vi "Config-Chan-SMU-Sweep.vi"(0 "VISA session":refnum<visa-resource-name>, 1 "function":i32(slide) max=4 scale=0.0..4.0, 2 "I name (max 6 chars)":string, 5 "unit to configure":i32(slide) max=5 scale=0.0..5.0, 7 "series resistance *":i32(slide) max=3 scale=0.0..3.0, 9 "standby":bool, 11 "error in (no error)":errorcluster, 12 "mode":i32(slide) max=4 scale=0.0..4.0, 13 "V name (max 6 chars)":string) -> (4 "VISA resource name out":refnum<visa-resource-name>, 15 "error out":errorcluster)   [LabVIEW 2016, in "Agilent 415X Series.lvlib"]
doc: "This VI configures an SMU for SWEEP mode measurement. \n\nThis VI corresponds to the Channel Definition Page of the instrument (when Measurement Mode is SWEEP). In general, it allows every setting change that can be made via the instrument's front panel although the change may cause a setting conflict when a measurement is initialied. This VI doesnot allow (by reporting an error) setting changes that can not be made via the instrument's front panel. For example, you may not set Series Resistance for units other than SMU1, SMU2/5.\n\n** The instrument used in the development of this instrument driver does not have an Expander Unit installed. Therefore commands related to SMU5/6 have not been verified."
uses:
  Agilent 415X Series.lvlib
panel:
  # "<--->"
  # "*   The Series Resistance control is active only if UnitToConfigure is SMU1 or SMU2/SMU5 (see description)\n** This VI does NOT report all setting errors.  Error checking must be done when a measurement is initialized."
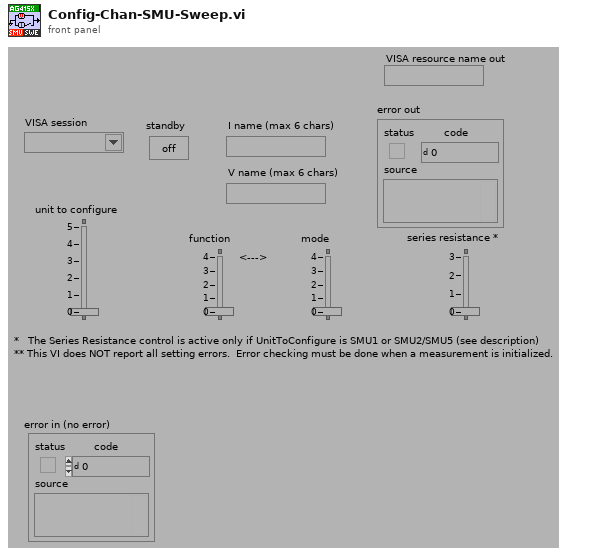
[diagram p1: front panel]
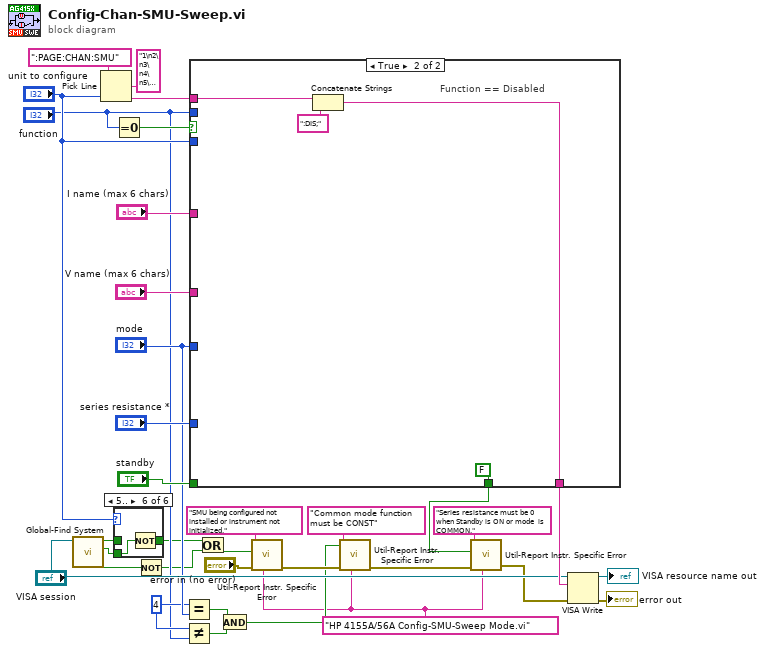
[diagram p0: block diagram]
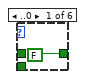
[diagram p2: hidden frame]
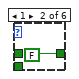
[diagram p3: hidden frame]
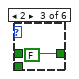
[diagram p4: hidden frame]
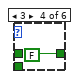
[diagram p5: hidden frame]
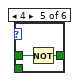
[diagram p6: hidden frame]
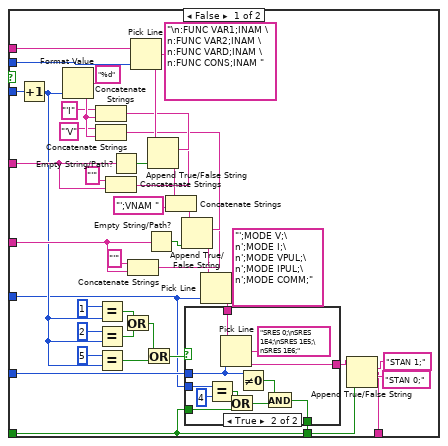
[diagram p7: hidden frame]
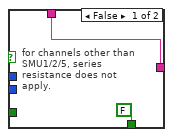
[diagram p8: hidden frame]
diagram:
  w12 = 4
  w8 = "HP 4155A/56A Config-SMU-Sweep Mode.vi"
  n1 = call "Global-Find System.vi"("VISA session"="VISA session") -> ("found"=w3:bool, "SMU6 present"=w24:bool, "SMU5 present"=w18:bool)  [unwired: 3 in, 5 out]
  n2 = Pick Line(string ("")=":PAGE:CHAN:SMU", multi-line string="1\n2\n3\n4\n5\n6", line index="unit to configure") -> (output string=w32:string)
  n3 = Equal To 0?(x="function") -> (x = 0?=w26:bool)
  n4 = case shown="5.." "unit to configure" {
    tunnel: [FALSE FALSE FALSE FALSE w40 w42] -> w4
    tunnel: w24 -> [_ _ _ _ _ w41]
    tunnel: w18 -> [_ _ _ _ w39 _]
    frame ..0 {
    }
    frame 1 {
    }
    frame 2 {
    }
    frame 3 {
    }
    frame 4 {
      n5 = Not(x=w39) -> (.not. x?=w40:bool)
    }
    frame 5.. {
      n6 = Not(x=w41) -> (.not. x?=w42:bool)
    }
  }
  n7 = Not(x=w3) -> (.not. x?=w2:bool)
  n8 = Equal?(x=w12, y="mode") -> (x = y?=w16:bool)
  n9 = Not Equal?(x=w12, y="function") -> (x != y?=w15:bool)
  n10 = case shown="True" w26 {
    tunnel: w32 -> [w83 w101]
    tunnel: "function" -> [w80 _]
    tunnel: "unit to configure" -> [w49 _]
    tunnel: "I name (max 6 chars)" -> [w74 _]
    tunnel: "V name (max 6 chars)" -> [w65 _]
    tunnel: "mode" -> [w44 _]
    tunnel: "series resistance *" -> [w58 _]
    tunnel: "standby" -> [w45 _]
    tunnel: [w46 w99] -> w28
    tunnel: [w43 FALSE] -> w6
    frame False {
      n11 = Increment(x=w49) -> (x+1=w47:i32)
      n12 = Format Value(format string="%d", value (0)=w47) -> (output string=w78:string)  [unwired: 1 in]
      n13 = Concatenate Strings("'I", w78) -> (w75:string)
      n14 = Concatenate Strings("'V", w78) -> (w68:string)
      n15 = Equal?(x=1, y=w47) -> (x = y?=w54:bool)
      n16 = Equal?(x=2, y=w47) -> (x = y?=w53:bool)
      n17 = Equal?(x=5, y=w47) -> (x = y?=w52:bool)
      n18 = Concatenate Strings("'", w74) -> (w72:string)
      n19 = Empty String/Path?(string/path=w74) -> (empty?=w81:bool)
      n20 = Or(x=w54, y=w53) -> (x .or. y?=w51:bool)
      n21 = Concatenate Strings("'", w65) -> (w64:string)
      n22 = Pick Line(string ("")=w83, multi-line string="\n:FUNC VAR1;INAM \n:FUNC VAR2;INAM \n:FUNC VARD;INAM \n:FUNC CONS;INAM ", line index=w80) -> (output string=w82:string)
      n23 = Or(x=w51, y=w52) -> (x .or. y?=w50:bool)
      n24 = Empty String/Path?(string/path=w65) -> (empty?=w67:bool)
      n25 = Append True/False String(1:w81, 2:w72, 3:w75, 4:w82) -> (0:w71:string)
      n26 = Concatenate Strings(w71, "';VNAM ") -> (w69:string)
      n27 = Append True/False String(1:w67, 2:w64, 3:w68, 4:w69) -> (0:w62:string)
      n28 = Pick Line(string ("")=w62, multi-line string="';MODE V;\n';MODE I;\n';MODE VPUL;\n';MODE IPUL;\n';MODE COMM;", line index=w44) -> (output string=w59:string)
      n29 = case shown="True" w50 {
        tunnel: w59 -> [w86 w96]
        tunnel: w58 -> [_ w89]
        tunnel: [w86 w95] -> w57
        tunnel: w45 -> [_ w92]
        tunnel: w44 -> [_ w94]
        tunnel: [FALSE w87] -> w43
        frame False {
          # "for channels other than\nSMU1/2/5, series \nresistance does not \napply."
        }
        frame True {
          n30 = Equal?(x=w94, y=4) -> (x = y?=w91:bool)
          n31 = Pick Line(string ("")=w96, multi-line string="SRES 0;\nSRES 1E4;\nSRES 1E5;\nSRES 1E6;", line index=w89) -> (output string=w95:string)
          n32 = Or(x=w91, y=w92) -> (x .or. y?=w90:bool)
          n33 = Not Equal To 0?(x=w89) -> (x != 0?=w88:bool)
          n34 = And(x=w88, y=w90) -> (x .and. y?=w87:bool)
        }
      }
      n35 = Append True/False String(1:w45, 2:"STAN 0;", 3:"STAN 1;", 4:w57) -> (0:w46:string)
    }
    frame True {
      # "Function == Disabled"
      n36 = Concatenate Strings(w101, ":DIS;") -> (w99:string)
    }
  }
  n37 = Or(x=w4, y=w2) -> (x .or. y?=w21:bool)
  n38 = And(x=w16, y=w15) -> (x .and. y?=w14:bool)
  n39 = call "Util-Report Instr. Specific Error.vi"("source"=w8, "error in (no error)"="error in (no error)", "error message"="SMU being configured not installed or instrument not initialized.", "new error"=w21) -> ("error out"=w20:errorcluster)  [unwired: 6 in, 1 out]
  n40 = call "Util-Report Instr. Specific Error.vi"("source"=w8, "error in (no error)"=w20, "error message"="Common mode function must be CONST", "new error"=w14) -> ("error out"=w9:errorcluster)  [unwired: 6 in, 1 out]
  n41 = call "Util-Report Instr. Specific Error.vi"("source"=w8, "error in (no error)"=w9, "error message"="Series resistance must be 0 when Standby is ON or mode  is COMMON.", "new error"=w6) -> ("error out"=w5:errorcluster)  [unwired: 6 in, 1 out]
  n42 = VISA Write(VISA resource name="VISA session", write buffer=w28, error in (no error)=w5) -> (VISA resource name out=→"VISA resource name out":refnum<visa-resource-name>, error out=→"error out":errorcluster)  [unwired: 1 out]
